vi "BeamTableEditor.vi"() -> ()   [LabVIEW 2021]
uses:
  D:/tmytek/Source/bbox-api/windows example/BBoxOne Series/LabVIEW/BBoxAPI.dll
  BBoxAPI.dll
  kernel32.dll
panel:
  in  "RX Beam Pattern":bool
  in  "RX beamId :\nRange from\n1 to 64":i32=1 min=1 max=64 step=1
  in  "RX_MIN_GAIN\nto\nRX_MAX_GAIN":dbl step=0.5
  in  "RX Theta \nRange from\n0 to 45":i32 min=0 max=45 step=1
  in  "RX Phi :\nRange from\n0 to 359":i32 min=0 max=359 step=1
  out "RX Store Beam Return":i32(ring) items=["OK"=0, "WARNING"=1, "ERROR"=2, "NO_RESPONSE"=3, "ERROR_GET_SN"=10, "ERROR_DEV_TYPE"=11, "ERROR_INIT_OBJECT"=12, "ERROR_DEV_NOT_INIT"=13, "ERROR_METHOD_NOT_FOUND"=14, "ERROR_REFLECTION"=15, "ERROR_POWER"=16, "ERROR_SCAN_NOT_FOUND"=17, "ERROR_UNMATCH_RETURN_TYPE"=18, "ERROR_NETWORK_NOT_INIT"=20, "ERROR_NETWORK_INIT"=21, "ERROR_NETWORK_CONNECT_TIMEOUT"=22, "ERROR_DISCONNECT"=23, "ERROR_SOCKET"=24, "ERROR_SEND_CMD"=25, "ERROR_RESP_CMD"=26, "ERROR_DEV_COUNT_ZERO"=30, "ERROR_DEV_DUMMY_FUNC"=31, "ERROR_CMD"=40, "ERROR_CMD_INIT"=41, "ERROR_BF_AAKIT"=100, "ERROR_BF_NO_AAKIT"=101, "ERROR_BF_CALI_PATH"=102, "ERROR_BF_BEAMXY"=103, "ERROR_BF_GEN"=104, "ERROR_BF_TRMODE"=105, "STATUS_BF_LOAD_CALI_INCOMPLTE"=106, "ERROR_BF_LOAD_CALI_PARSE_FAILED"=107, "ERROR_BF_UNLOAD_CALI"=108, "ERROR_BF_CALI_VERSION_UNSUPPORTED"=109, "ERROR_BF_CALI_DATA_NOT_FOUND"=110, "ERROR_FREQ_EQUATION"=250, "ERROR_PLO_CRC"=251, "WARNING_HARMONIC"=252, "ERROR_HARMONIC_BLOCK"=253, "ERROR_FW_UPGRADE_IP_INVALID"=300, "ERROR_FW_VERSION_NOT_SUPPORT"=301]
  out "getFrequencyList":string[](array[string])
  out "SN":string
  out "current state":i32
  out "ScanningDevice":string[](array[string])
  out "Target SN":string
  in  "Device SN":string="B00000000-00"
  out "SN_is_match":bool
  out "Init":i32(ring) items=["OK"=0, "WARNING"=1, "ERROR"=2, "NO_RESPONSE"=3, "ERROR_GET_SN"=10, "ERROR_DEV_TYPE"=11, "ERROR_INIT_OBJECT"=12, "ERROR_DEV_NOT_INIT"=13, "ERROR_METHOD_NOT_FOUND"=14, "ERROR_REFLECTION"=15, "ERROR_POWER"=16, "ERROR_SCAN_NOT_FOUND"=17, "ERROR_UNMATCH_RETURN_TYPE"=18, "ERROR_NETWORK_NOT_INIT"=20, "ERROR_NETWORK_INIT"=21, "ERROR_NETWORK_CONNECT_TIMEOUT"=22, "ERROR_DISCONNECT"=23, "ERROR_SOCKET"=24, "ERROR_SEND_CMD"=25, "ERROR_RESP_CMD"=26, "ERROR_DEV_COUNT_ZERO"=30, "ERROR_DEV_DUMMY_FUNC"=31, "ERROR_CMD"=40, "ERROR_CMD_INIT"=41, "ERROR_BF_AAKIT"=100, "ERROR_BF_NO_AAKIT"=101, "ERROR_BF_CALI_PATH"=102, "ERROR_BF_BEAMXY"=103, "ERROR_BF_GEN"=104, "ERROR_BF_TRMODE"=105, "STATUS_BF_LOAD_CALI_INCOMPLTE"=106, "ERROR_BF_LOAD_CALI_PARSE_FAILED"=107, "ERROR_BF_UNLOAD_CALI"=108, "ERROR_BF_CALI_VERSION_UNSUPPORTED"=109, "ERROR_BF_CALI_DATA_NOT_FOUND"=110, "ERROR_FREQ_EQUATION"=250, "ERROR_PLO_CRC"=251, "WARNING_HARMONIC"=252, "ERROR_HARMONIC_BLOCK"=253, "ERROR_FW_UPGRADE_IP_INVALID"=300, "ERROR_FW_VERSION_NOT_SUPPORT"=301]
  out "checkCaliTableLocation":bool
  out "Console Log":string
  in  "Target Freq Index":i32 min=1 max=2 step=1
  out "setOperatingFreq":i32(ring)=2 items=["OK"=0, "WARNING"=1, "ERROR"=2, "NO_RESPONSE"=3, "ERROR_GET_SN"=10, "ERROR_DEV_TYPE"=11, "ERROR_INIT_OBJECT"=12, "ERROR_DEV_NOT_INIT"=13, "ERROR_METHOD_NOT_FOUND"=14, "ERROR_REFLECTION"=15, "ERROR_POWER"=16, "ERROR_NETWORK_NOT_INIT"=20, "ERROR_NETWORK_INIT"=21, "ERROR_NETWORK_CONNECT_TIMEOUT"=22, "ERROR_DISCONNECT"=23, "ERROR_SOCKET"=24, "ERROR_SEND_CMD"=25, "ERROR_RESP_CMD"=26, "ERROR_DEV_COUNT_ZERO"=30, "ERROR_CMD"=40, "ERROR_CMD_INIT"=41, "ERROR_BF_AAKIT"=100, "ERROR_BF_NO_AAKIT"=101, "ERROR_BF_CALI_PATH"=102, "ERROR_BF_BEAMXY"=103, "ERROR_BF_GEN"=104, "ERROR_BF_TRMODE"=105, "STATUS_BF_LOAD_CALI_INCOMPLTE"=106, "ERROR_BF_LOAD_CALI_PARSE_FAILED"=107, "ERROR_FREQ_EQUATION"=250, "ERROR_PLO_CRC"=251, "WARNING_HARMONIC"=252, "ERROR_HARMONIC_BLOCK"=253]
  out "TX_MIN_GAIN":dbl
  out "TX_MAX_GAIN":dbl
  out "RX_MIN_GAIN":dbl
  out "RX_MAX_GAIN":dbl
  out "getAAKitList":string[](array[string])
  out "selectAAKit":i32(ring)=2 items=["OK"=0, "WARNING"=1, "ERROR"=2, "NO_RESPONSE"=3, "ERROR_GET_SN"=10, "ERROR_DEV_TYPE"=11, "ERROR_INIT_OBJECT"=12, "ERROR_DEV_NOT_INIT"=13, "ERROR_METHOD_NOT_FOUND"=14, "ERROR_REFLECTION"=15, "ERROR_POWER"=16, "ERROR_NETWORK_NOT_INIT"=20, "ERROR_NETWORK_INIT"=21, "ERROR_NETWORK_CONNECT_TIMEOUT"=22, "ERROR_DISCONNECT"=23, "ERROR_SOCKET"=24, "ERROR_SEND_CMD"=25, "ERROR_RESP_CMD"=26, "ERROR_DEV_COUNT_ZERO"=30, "ERROR_CMD"=40, "ERROR_CMD_INIT"=41, "ERROR_BF_AAKIT"=100, "ERROR_BF_NO_AAKIT"=101, "ERROR_BF_CALI_PATH"=102, "ERROR_BF_BEAMXY"=103, "ERROR_BF_GEN"=104, "ERROR_BF_TRMODE"=105, "STATUS_BF_LOAD_CALI_INCOMPLTE"=106, "ERROR_BF_LOAD_CALI_PARSE_FAILED"=107, "ERROR_FREQ_EQUATION"=250, "ERROR_PLO_CRC"=251, "WARNING_HARMONIC"=252, "ERROR_HARMONIC_BLOCK"=253]
  out "RX Beam Table":string[][](array[string])
  out "TX Beam Table":string[][](array[string])
  in  "Target AAKit Index":i32 min=1 max=2 step=1
  out "Target AAKit Name":string
  in  "TX beamId :\nRange from\n1 to 64":i32=1 min=1 max=64 step=1
  in  "TX_MIN_GAIN\nto\nTX_MAX_GAIN":dbl step=0.5
  in  "TX Theta \nRange from\n0 to 45":i32 min=0 max=45 step=1
  in  "TX Phi :\nRange from\n0 to 359":i32 min=0 max=359 step=1
  out "TX Store Beam Return":i32(ring) items=["OK"=0, "WARNING"=1, "ERROR"=2, "NO_RESPONSE"=3, "ERROR_GET_SN"=10, "ERROR_DEV_TYPE"=11, "ERROR_INIT_OBJECT"=12, "ERROR_DEV_NOT_INIT"=13, "ERROR_METHOD_NOT_FOUND"=14, "ERROR_REFLECTION"=15, "ERROR_POWER"=16, "ERROR_SCAN_NOT_FOUND"=17, "ERROR_UNMATCH_RETURN_TYPE"=18, "ERROR_NETWORK_NOT_INIT"=20, "ERROR_NETWORK_INIT"=21, "ERROR_NETWORK_CONNECT_TIMEOUT"=22, "ERROR_DISCONNECT"=23, "ERROR_SOCKET"=24, "ERROR_SEND_CMD"=25, "ERROR_RESP_CMD"=26, "ERROR_DEV_COUNT_ZERO"=30, "ERROR_DEV_DUMMY_FUNC"=31, "ERROR_CMD"=40, "ERROR_CMD_INIT"=41, "ERROR_BF_AAKIT"=100, "ERROR_BF_NO_AAKIT"=101, "ERROR_BF_CALI_PATH"=102, "ERROR_BF_BEAMXY"=103, "ERROR_BF_GEN"=104, "ERROR_BF_TRMODE"=105, "STATUS_BF_LOAD_CALI_INCOMPLTE"=106, "ERROR_BF_LOAD_CALI_PARSE_FAILED"=107, "ERROR_BF_UNLOAD_CALI"=108, "ERROR_BF_CALI_VERSION_UNSUPPORTED"=109, "ERROR_BF_CALI_DATA_NOT_FOUND"=110, "ERROR_FREQ_EQUATION"=250, "ERROR_PLO_CRC"=251, "WARNING_HARMONIC"=252, "ERROR_HARMONIC_BLOCK"=253, "ERROR_FW_UPGRADE_IP_INVALID"=300, "ERROR_FW_VERSION_NOT_SUPPORT"=301]
  in  "Program Stop":bool
  in  "TX Beam Pattern":bool
  out "Exists Table Filenames":string[](array[string])
  out "Get Current Working Directory":path
  in  "Set Current Working Directory":path
  in  "Start":bool
  # "Notice:\n\n1.  User can directly edit the beam settings (beamId, mode, db, theta, phi) and run the program to store beam pattern.\n\n     1.1 Store beam pattern and then read all beam patterns to GUI.\n\n\n2. Beam gain range definition is as below\n\n      2.1 Dynamic range of TX mode contains TX_MIN_GAIN and TX_MAX_GAIN read from calibration table.\n\n      2.2 TX beam gain setting must less than or equal to TX_MAX_GAIN and larger than or equal to TX_MIN_GAIN.\n\n      2.3 Dynamic range of RX mode contains RX_MIN_GAIN and RX_MAX_GAIN read from the calibration table.\n\n      2.4 RX beam gain setting must less than or equal to RX_MAX_GAIN and larger than or equal to RX_MIN_GAIN.\n\n\n3. Beam Id range is from 1 to 64.\n\n\n4. TX mode equals to 1 and RX mode equals to 2.\n\n\n5. Theta range is  from 0 to 45.\n\n\n6. Phi range is from 0 to 359.\n\n\n7. The right side beam tables  are readonly.\n\n     7.1 The  table column definition is [ beamId, mode, db, theta, phi ]"
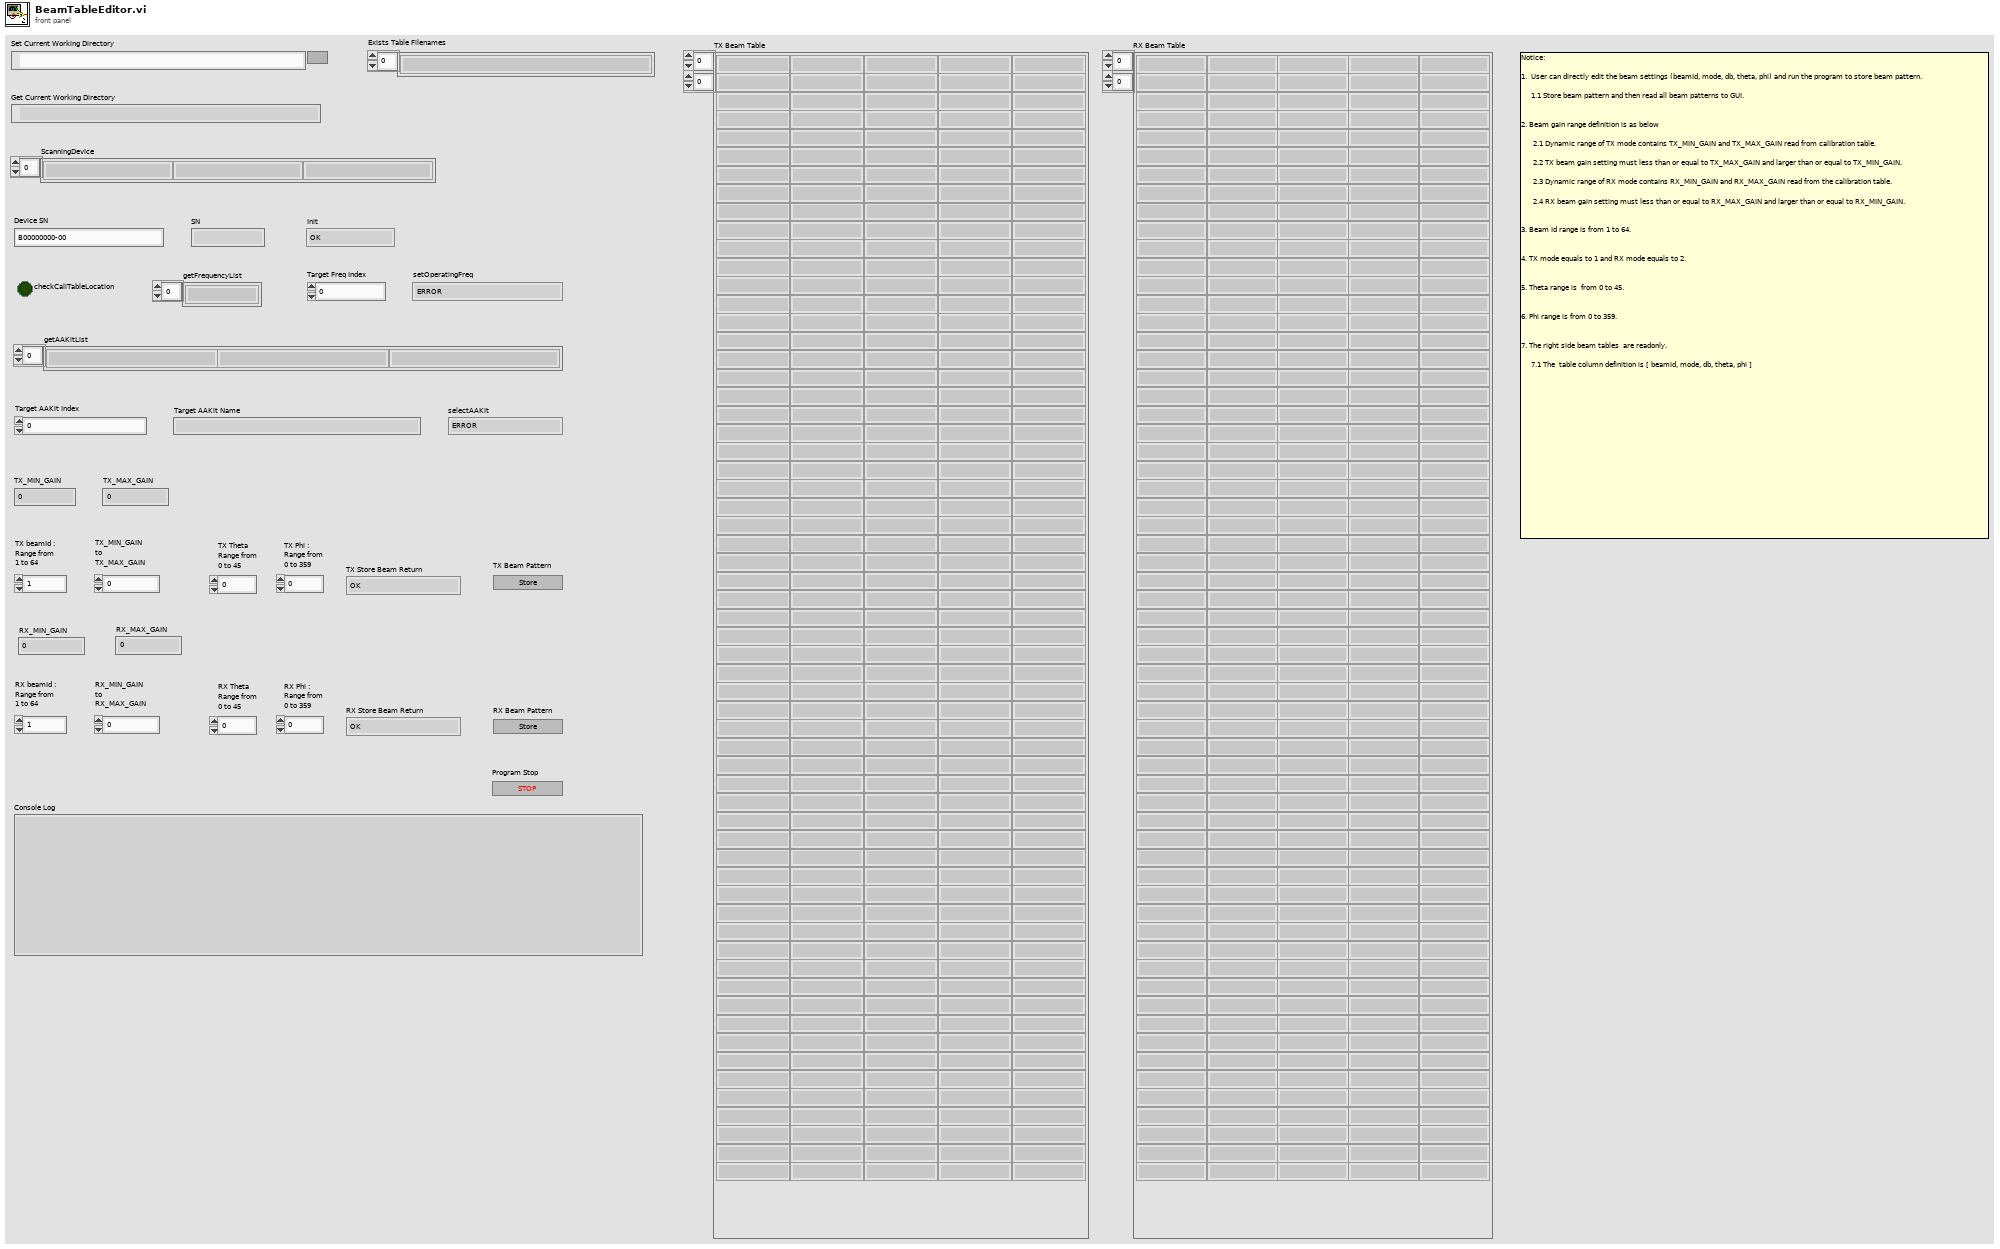
[diagram p1: front panel]
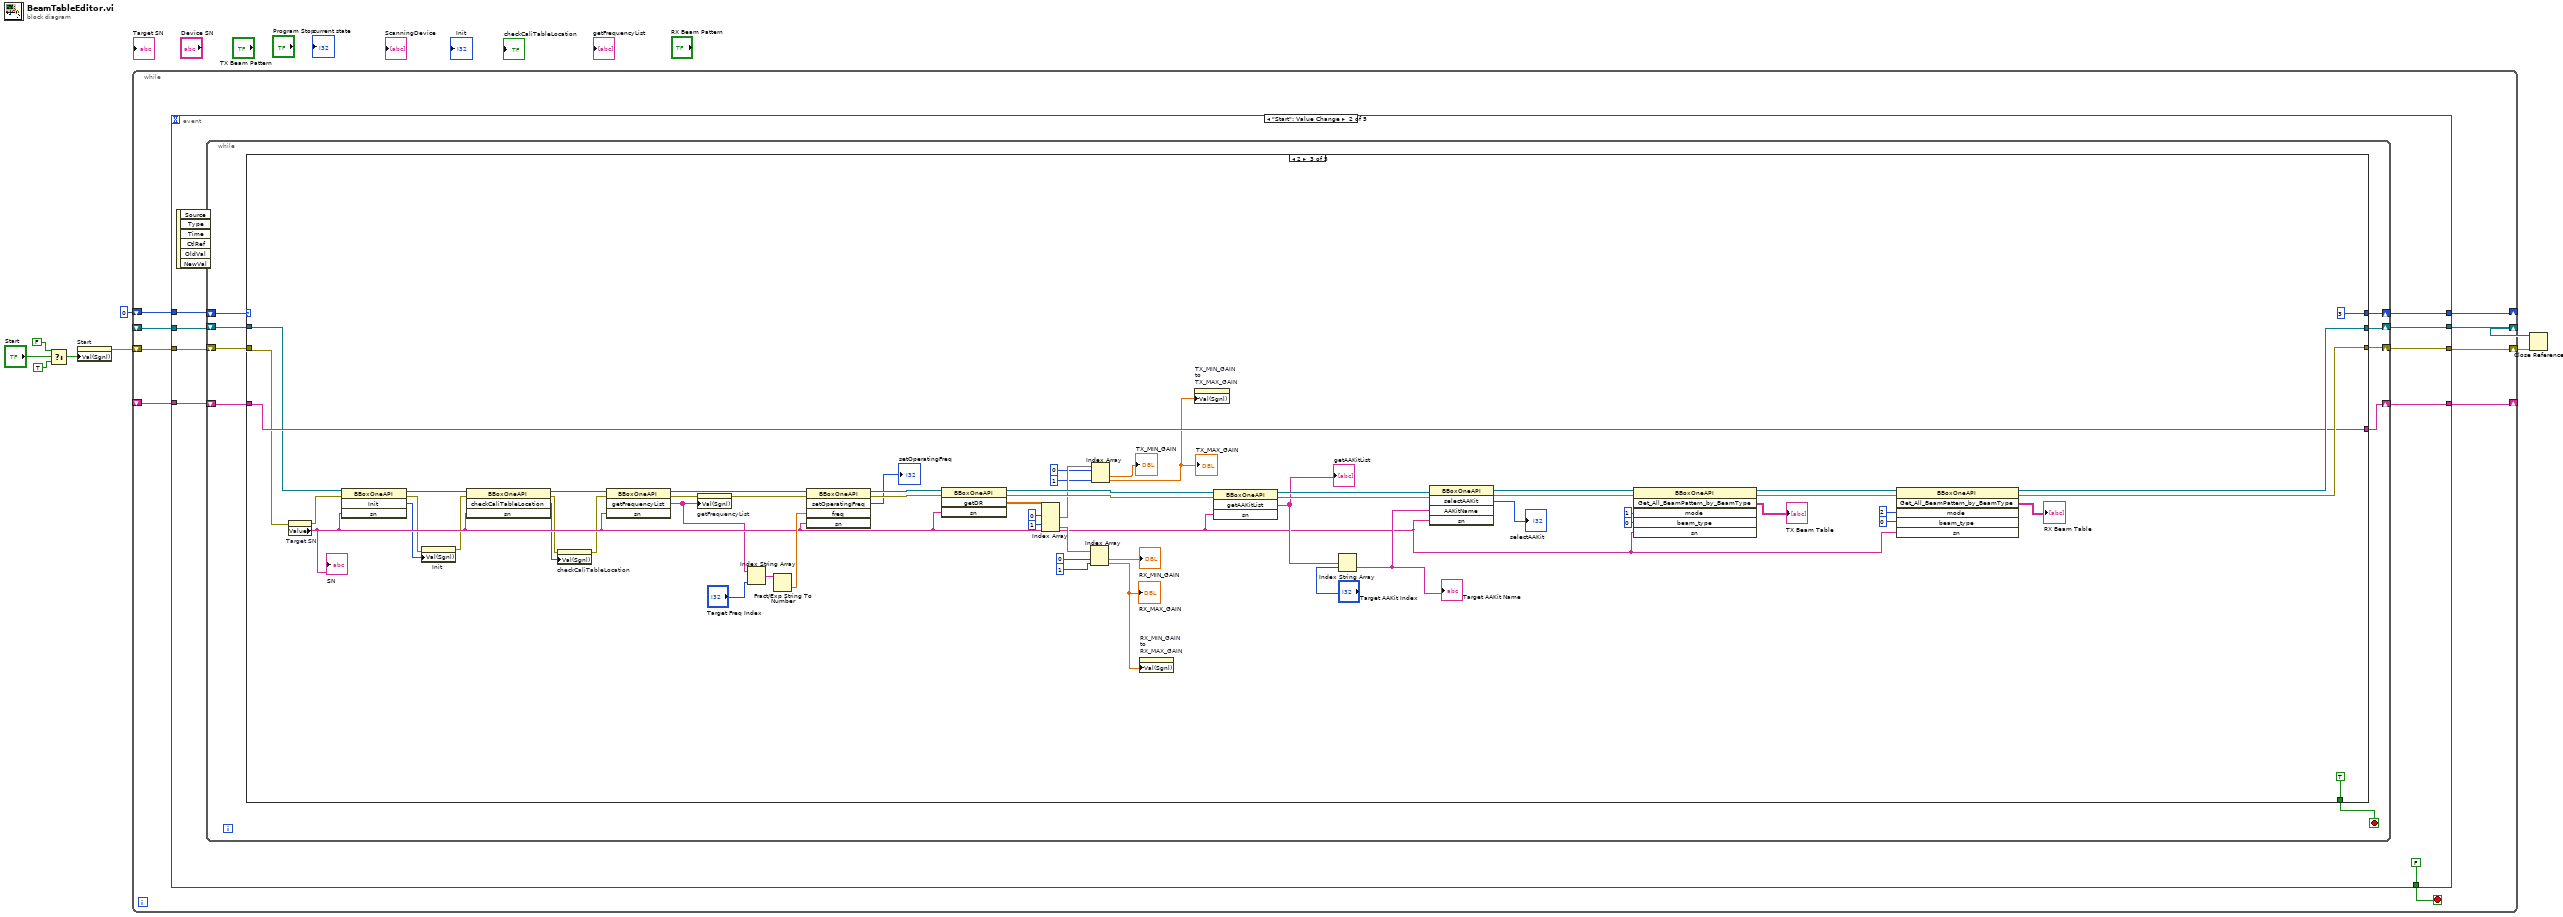
[diagram p0: block diagram]
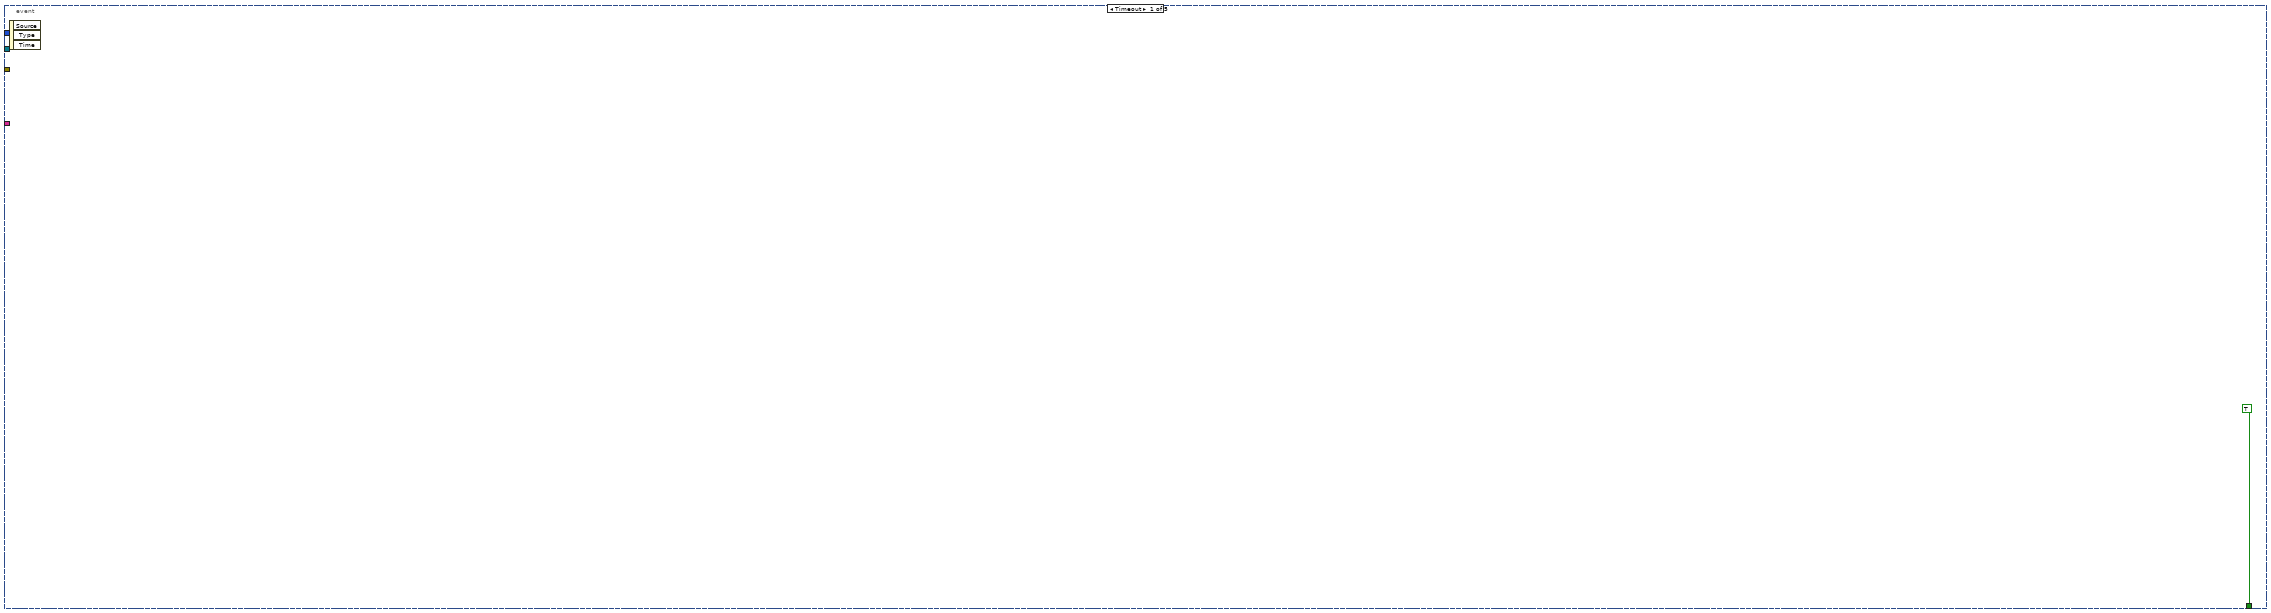
[diagram p2: hidden frame]
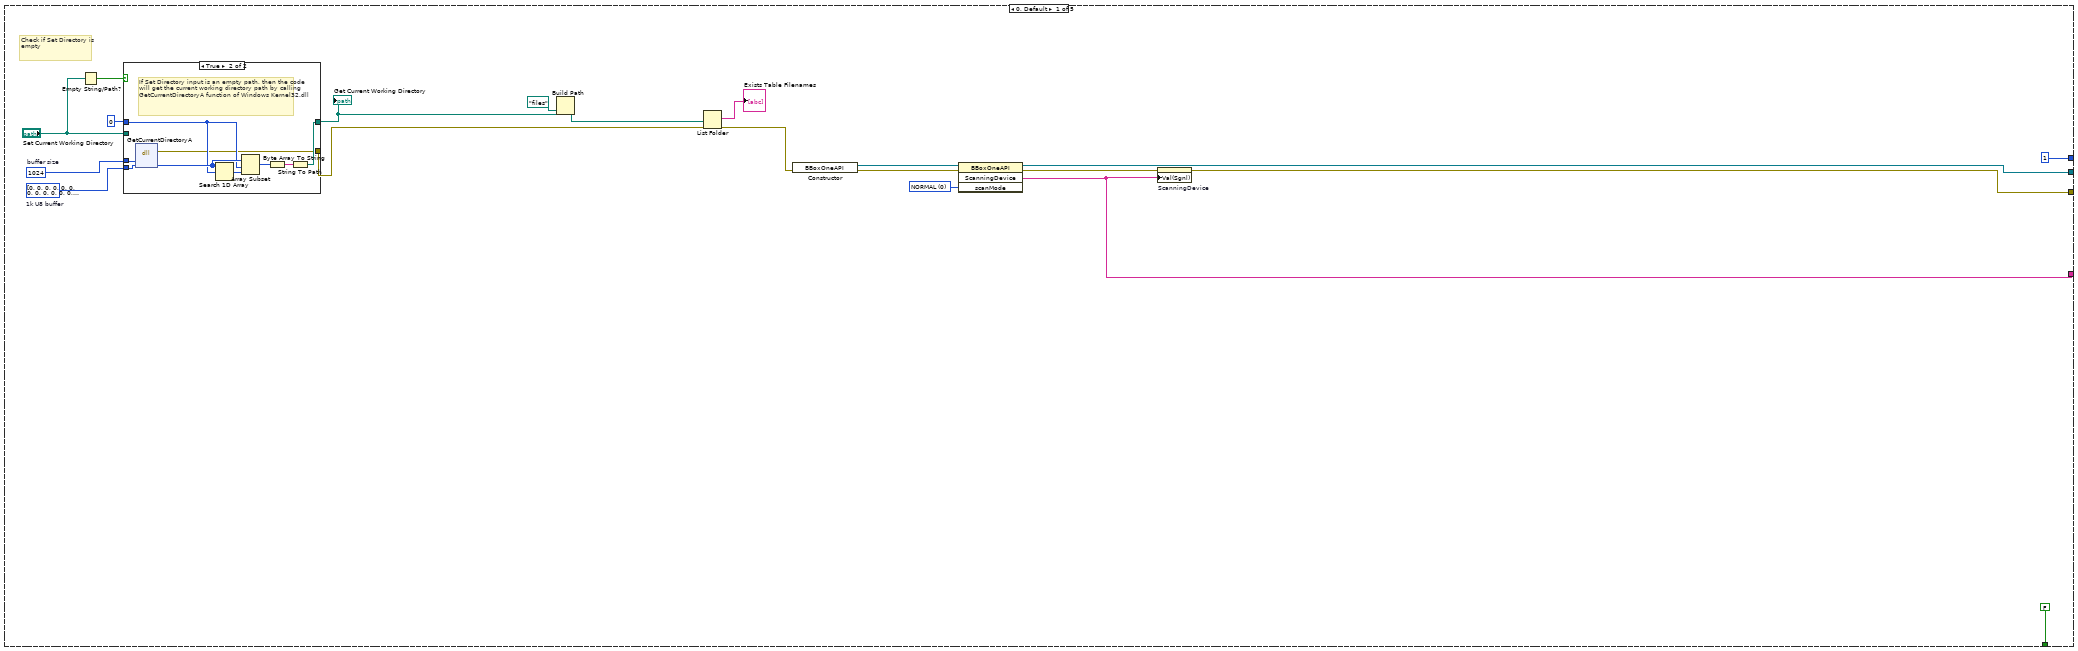
[diagram p3: hidden frame]
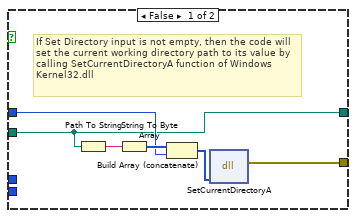
[diagram p4: hidden frame]
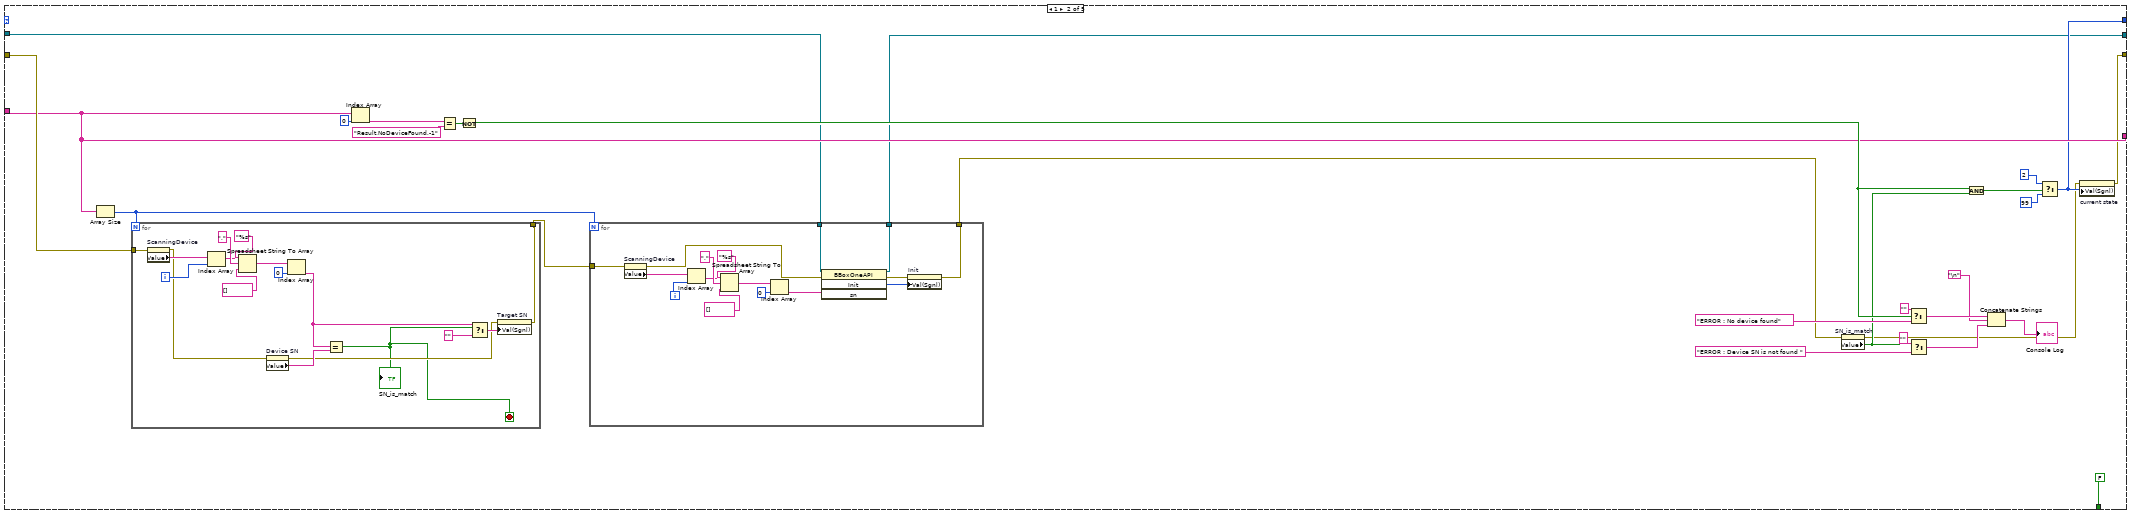
[diagram p5: hidden frame]
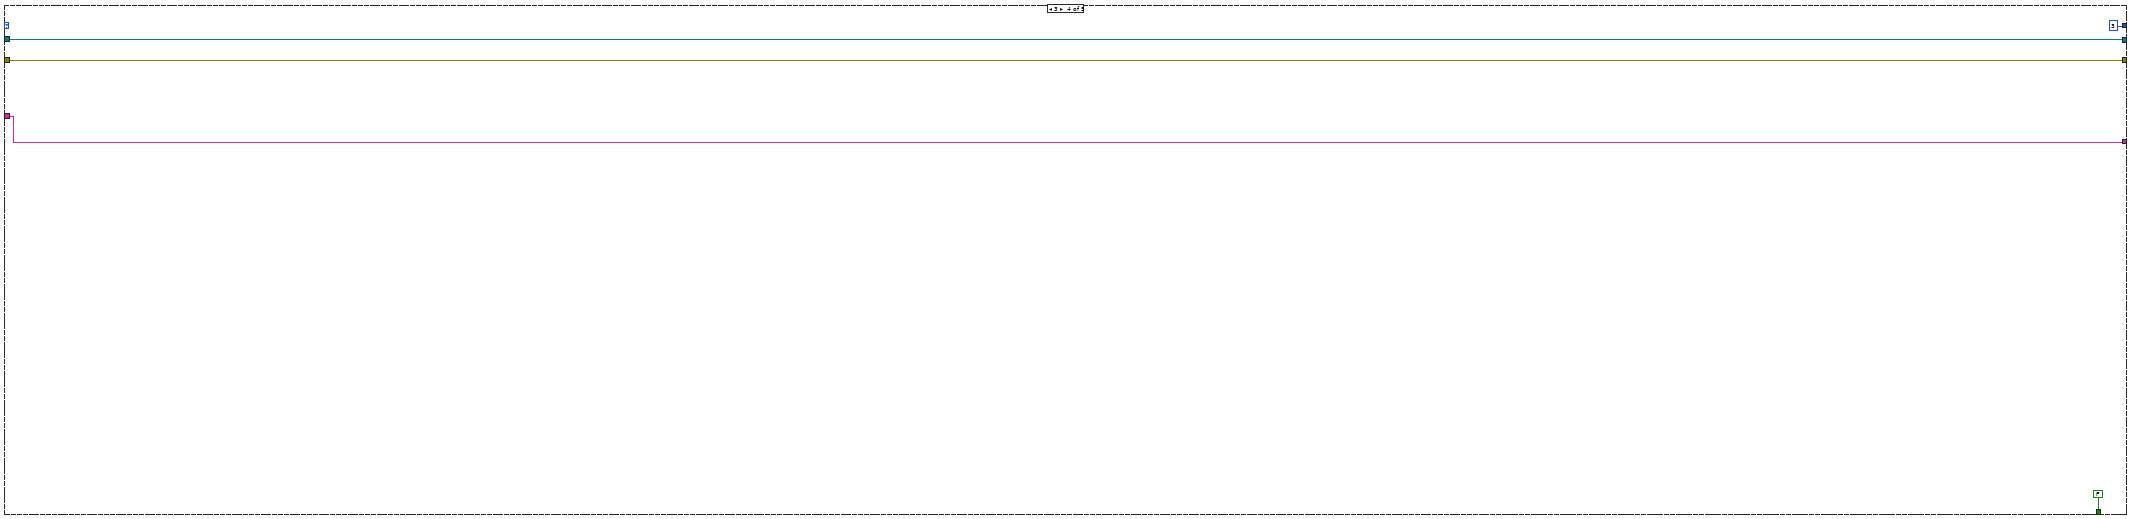
[diagram p6: hidden frame]
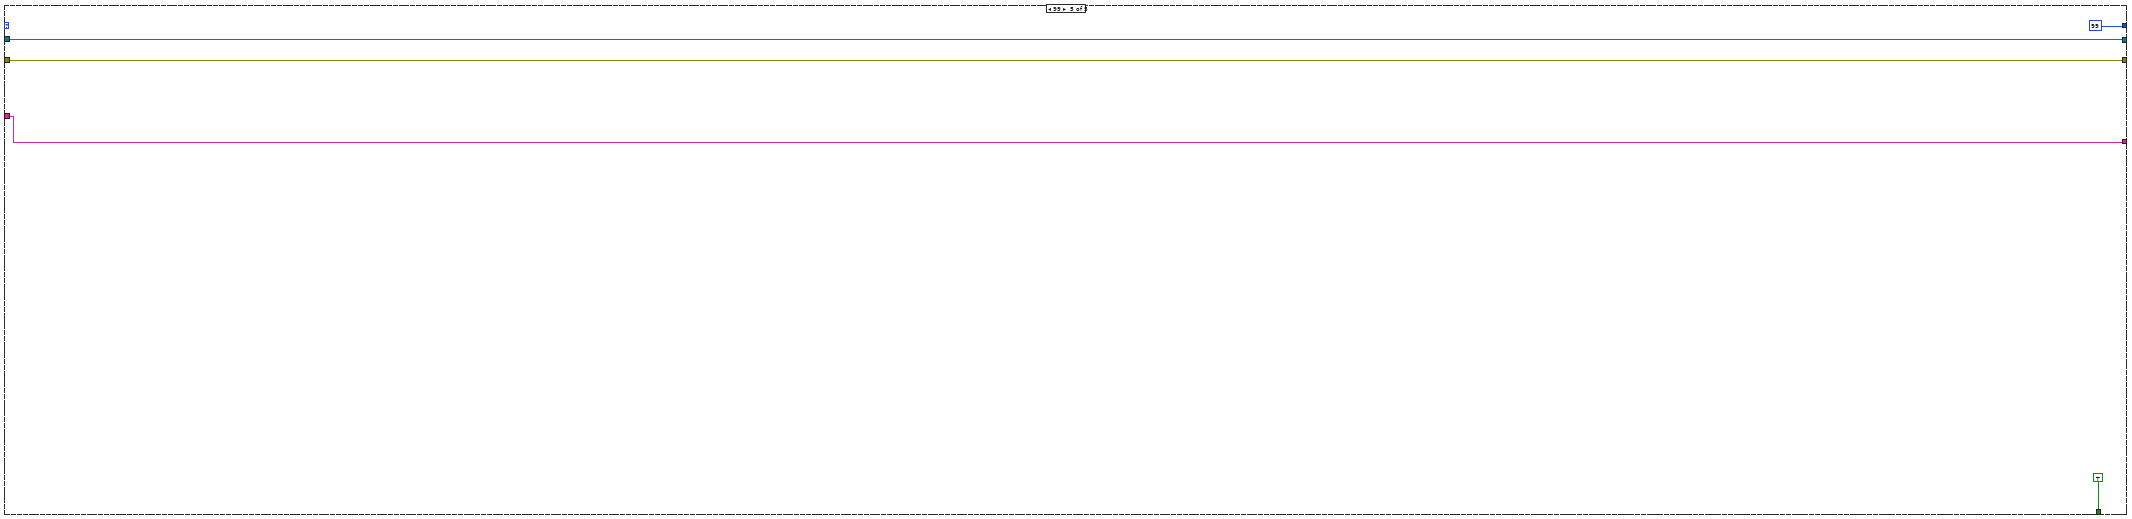
[diagram p7: hidden frame]
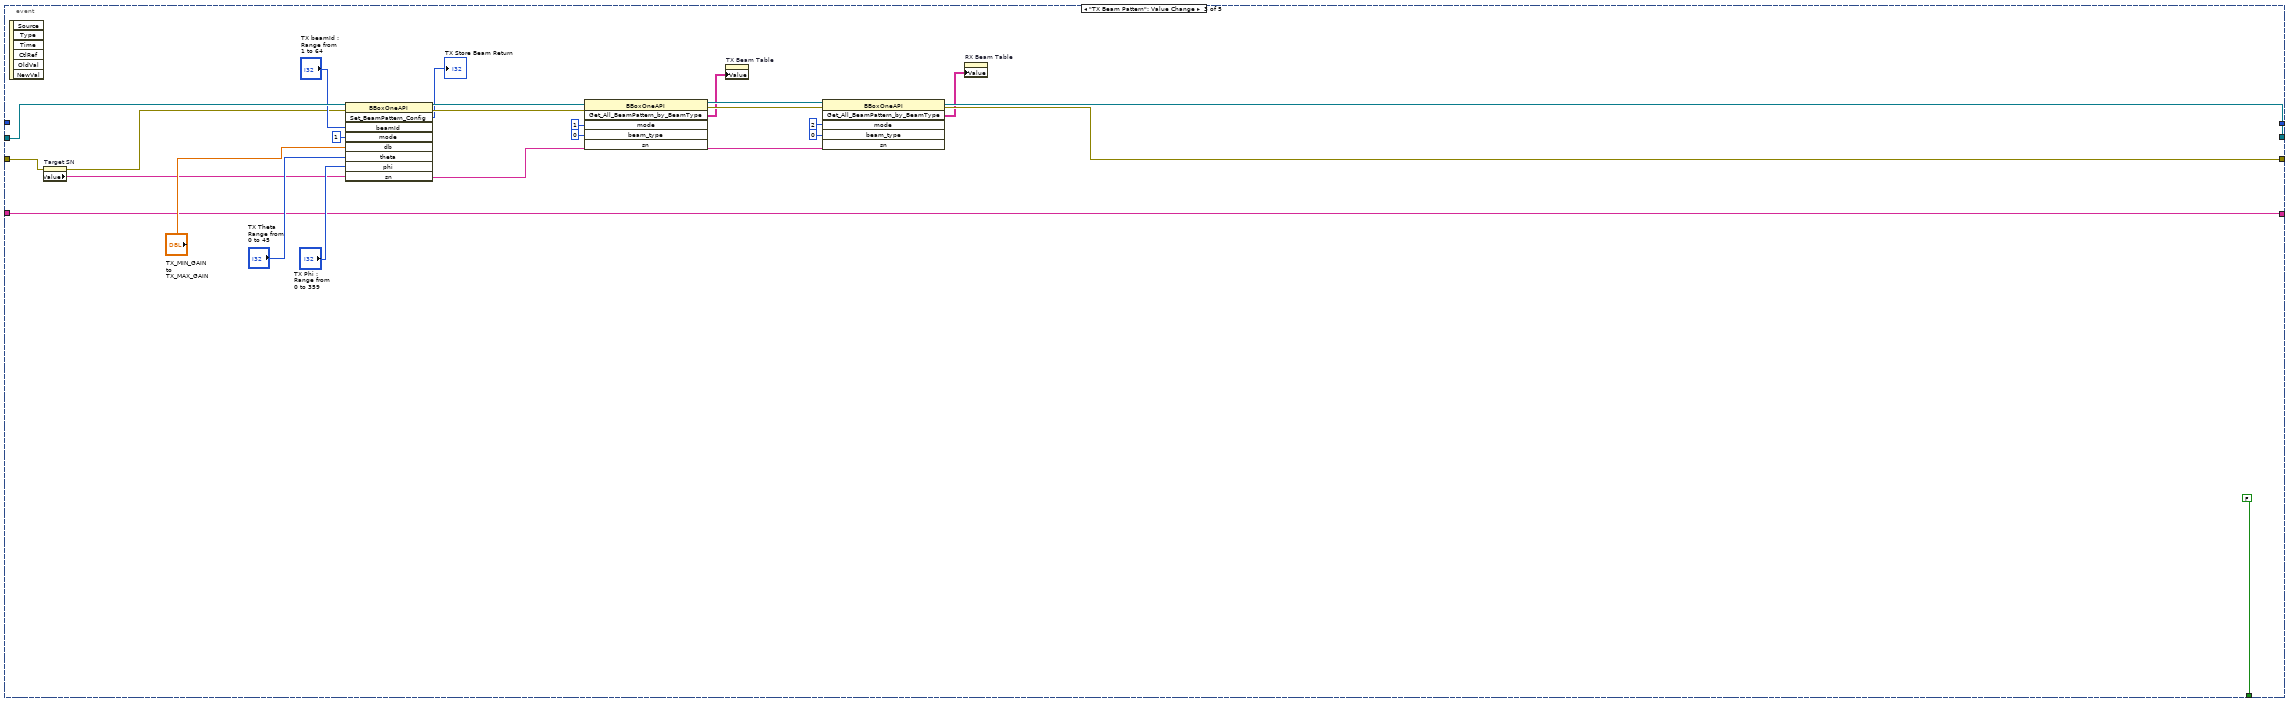
[diagram p8: hidden frame]
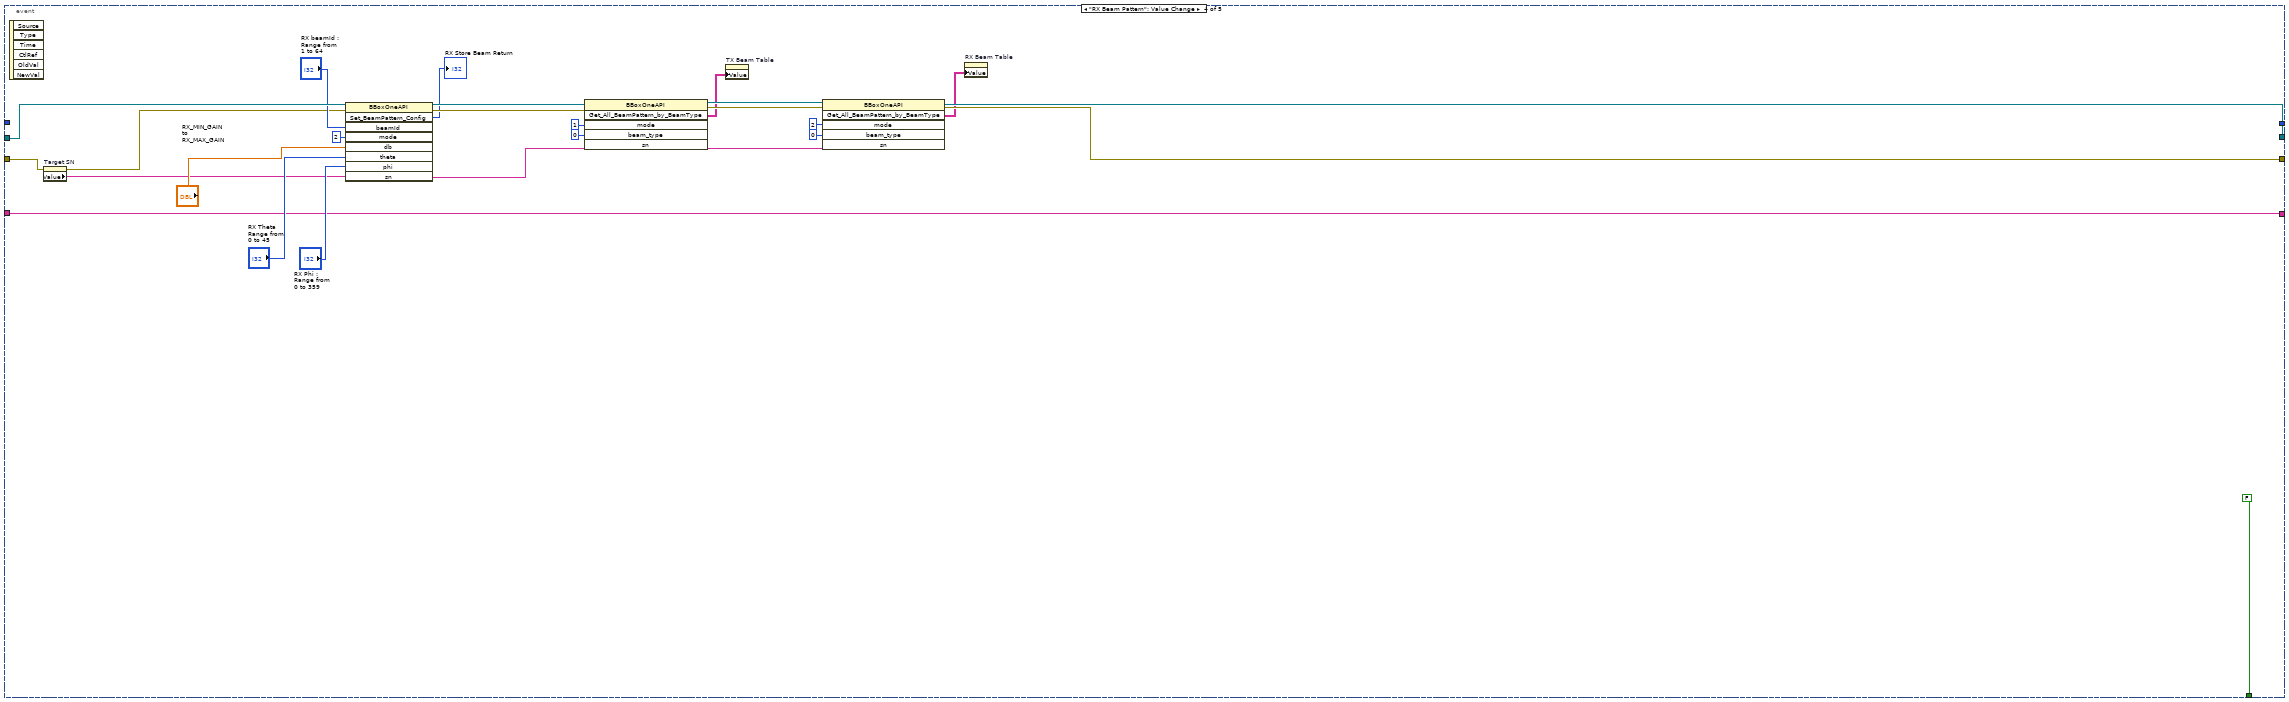
[diagram p9: hidden frame]
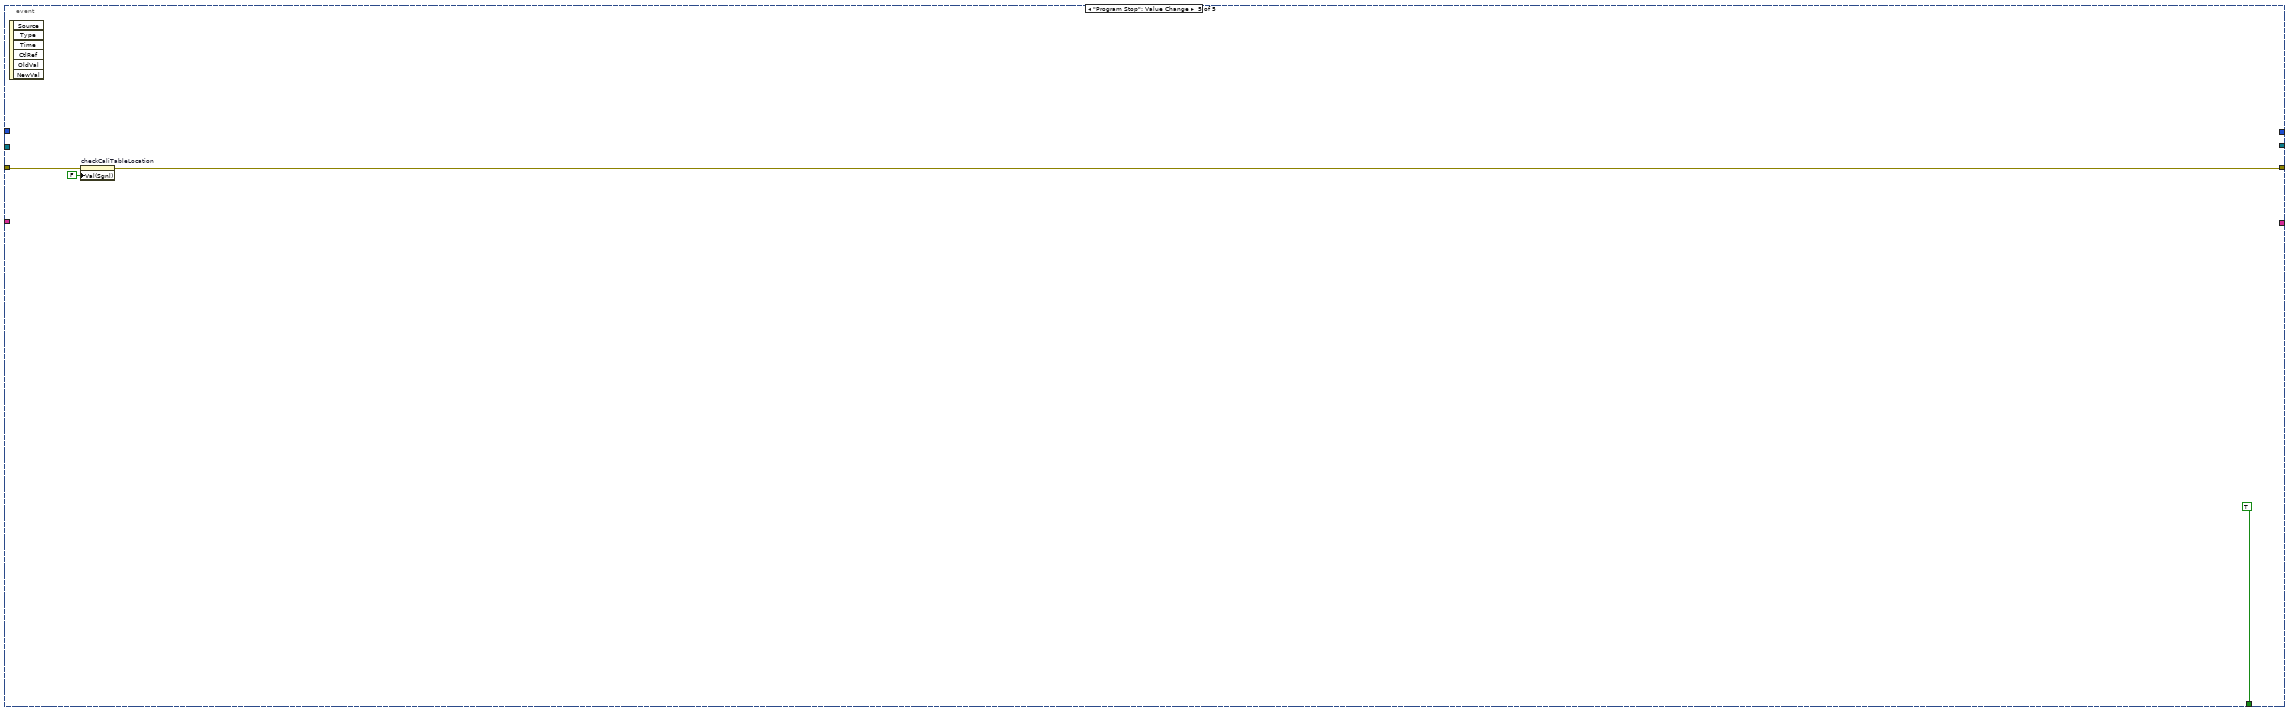
[diagram p10: hidden frame]
diagram:
  n1 = Select(t=FALSE, s="Start", f=TRUE) -> (s? t:f=w6:bool)
  n2 = property on="Start" class="Bool (strict)"("Val(Sgnl)"=w6) -> (error out=w3:errorcluster)  [unwired: 2 in, 1 out]
  n3 = while {
    shift-right: [w16] -> w8
    shift-left: _ -> [w14]
    shift-right: [w15] -> w7
    shift-left: w3 -> [w13]
    shift-right: [w12] -> _
    shift-left: _ -> [w11]
    shift-right: [w10] -> _
    shift-left: 0 -> [w9]
    stop <- w17 stop-if-true
    n4 = event shown="[1] \"Start\": Value Change" {
      selector: _ -> [_ _ _ _ _]
      dyn-events: _ -> [_ _ _ _ _]
      timeout: _ -> [_ _ _ _ _]
      tunnel: [TRUE FALSE FALSE FALSE TRUE] -> w17
      tunnel: [_ w27 w214 w238 _] -> w16
      tunnel: [_ w26 w213 w237 w249] -> w15
      tunnel: w14 -> [_ w25 w223 w247 _]
      tunnel: w13 -> [_ w24 w203 w227 w251]
      tunnel: [_ w22 w205 w229 _] -> w12
      tunnel: w11 -> [_ w21 w205 w229 _]
      tunnel: [_ w20 _ _ _] -> w10
      tunnel: w9 -> [_ w19 _ _ _]
      event Timeout {
        n5 = event-data() -> ()  [unwired: 1 in, 3 out]
      }
      event "Start": Value Change {
        n6 = event-data() -> ()  [unwired: 1 in, 6 out]
        n7 = while {
          shift-right: [w36] -> w20
          shift-left: w19 -> [w28]
          shift-right: [w35] -> w27
          shift-left: w25 -> [w33]
          shift-right: [w34] -> w26
          shift-left: w24 -> [w32]
          shift-right: [w30] -> w22
          shift-left: w21 -> [w29]
          stop <- w31 stop-if-true
          n8 = case shown="2" w28 {
            tunnel: [w37 w81 w156 w194 w198] -> w34
            tunnel: [w41 w73 w157 w195 w197] -> w35
            tunnel: [1 w82 3 3 99] -> w36
            tunnel: [FALSE FALSE TRUE FALSE TRUE] -> w31
            tunnel: w33 -> [_ w74 w146 w195 w197]
            tunnel: w32 -> [_ w84 w150 w194 w198]
            tunnel: [w39 w83 w154 w193 w196] -> w30
            tunnel: w29 -> [_ w83 w154 w193 w196]
            frame 0, Default {
              w51 = 1024  # buffer size
              w56 = 0 items=["NORMAL", "FAST"] ("scanMode")
              w50 = u8[] [0, 0, 0, 0, 0, 0, 0, 0, 0, 0, 0, 0, 0, 0, 0, 0, 0, 0, 0, 0, 0, 0, 0, 0, 0, 0, 0, 0, 0, 0, 0, 0, 0, 0, 0, 0, 0, 0, 0, 0, 0, 0, 0, 0, 0, 0, 0, 0, 0, 0, 0, 0, 0, 0, 0, 0, 0, 0, 0, 0, 0, 0, 0, 0, 0, 0, 0, 0, 0, 0, 0, 0, 0, 0, 0, 0, 0, 0, 0, 0, 0, 0, 0, 0, 0, 0, 0, 0, 0, 0, 0, 0, 0, 0, 0, 0, 0, 0, 0, 0, 0, 0, 0, 0, 0, 0, 0, 0, 0, 0, 0, 0, 0, 0, 0, 0, 0, 0, 0, 0, 0, 0, 0, 0, 0, 0, 0, 0, 0, 0, 0, 0, 0, 0, 0, 0, 0, 0, 0, 0, 0, 0, 0, 0, 0, 0, 0, 0, 0, 0, 0, 0, 0, 0, 0, 0, 0, 0, 0, 0, 0, 0, 0, 0, 0, 0, 0, 0, 0, 0, 0, 0, 0, 0, 0, 0, 0, 0, 0, 0, 0, 0, 0, 0, 0, 0, 0, 0, 0, 0, 0, 0, 0, 0, 0, 0, 0, 0, 0, 0, 0, 0, 0, 0, 0, 0, 0, 0, 0, 0, 0, 0, 0, 0, 0, 0, 0, 0, 0, 0, 0, 0, 0, 0, 0, 0, 0, 0, 0, 0, 0, 0, 0, 0, 0, 0, 0, 0, 0, 0, 0, 0, 0, 0, 0, 0, 0, 0, 0, 0, 0, 0, 0, 0, 0, 0, 0, 0, 0, 0, 0, 0, 0, 0, 0, 0, 0, 0, 0, 0, 0, 0, 0, 0, 0, 0, 0, 0, 0, 0, 0, 0, 0, 0, 0, 0, 0, 0, 0, 0, 0, 0, 0, 0, 0, 0, 0, 0, 0, 0, 0, 0, 0, 0, 0, 0, 0, 0, 0, 0, 0, 0, 0, 0, 0, 0, 0, 0, 0, 0, 0, 0, 0, 0, 0, 0, 0, 0, 0, 0, 0, 0, 0, 0, 0, 0, 0, 0, 0, 0, 0, 0, 0, 0, 0, 0, 0, 0, 0, 0, 0, 0, 0, 0, 0, 0, 0, 0, 0, 0, 0, 0, 0, 0, 0, 0, 0, 0, 0, 0, 0, 0, 0, 0, 0, 0, 0, 0, 0, 0, 0, 0, 0, 0, 0, 0, 0, 0, 0, 0, 0, 0, 0, 0, 0, 0, 0, 0, 0, 0, 0, 0, 0, 0, 0, 0, 0, 0, 0, 0, 0, 0, 0, 0, 0, 0, 0, 0, 0, 0, 0, 0, 0, 0, 0, 0, 0, 0, 0, 0, 0, 0, 0, 0, 0, 0, 0, 0, 0, 0, 0, 0, 0, 0, 0, 0, 0, 0, 0, 0, 0, 0, 0, 0, 0, 0, 0, 0, 0, 0, 0, 0, 0, 0, 0, 0, 0, 0, 0, 0, 0, 0, 0, 0, 0, 0, 0, 0, 0, 0, 0, 0, 0, 0, 0, 0, 0, 0, 0, 0, 0, 0, 0, 0, 0, 0, 0, 0, 0, 0, 0, 0, 0, 0, 0, 0, 0, 0, 0, 0, 0, 0, 0, 0, 0, 0, 0, 0, 0, 0, 0, 0, 0, 0, 0, 0, 0, 0, 0, 0, 0, 0, 0, 0, 0, 0, 0, 0, 0, 0, 0, 0, 0, 0, 0, 0, 0, 0, 0, 0, 0, 0, 0, 0, 0, 0, 0, 0, 0, 0, 0, 0, 0, 0, 0, 0, 0, 0, 0, 0, 0, 0, 0, 0, 0, 0, 0, 0, 0, 0, 0, 0, 0, 0, 0, 0, 0, 0, 0, 0, 0, 0, 0, 0, 0, 0, 0, 0, 0, 0, 0, 0, 0, 0, 0, 0, 0, 0, 0, 0, 0, 0, 0, 0, 0, 0, 0, 0, 0, 0, 0, 0, 0, 0, 0, 0, 0, 0, 0, 0, 0, 0, 0, 0, 0, 0, 0, 0, 0, 0, 0, 0, 0, 0, 0, 0, 0, 0, 0, 0, 0, 0, 0, 0, 0, 0, 0, 0, 0, 0, 0, 0, 0, 0, 0, 0, 0, 0, 0, 0, 0, 0, 0, 0, 0, 0, 0, 0, 0, 0, 0, 0, 0, 0, 0, 0, 0, 0, 0, 0, 0, 0, 0, 0, 0, 0, 0, 0, 0, 0, 0, 0, 0, 0, 0, 0, 0, 0, 0, 0, 0, 0, 0, 0, 0, 0, 0, 0, 0, 0, 0, 0, 0, 0, 0, 0, 0, 0, 0, 0, 0, 0, 0, 0, 0, 0, 0, 0, 0, 0, 0, 0, 0, 0, 0, 0, 0, 0, 0, 0, 0, 0, 0, 0, 0, 0, 0, 0, 0, 0, 0, 0, 0, 0, 0, 0, 0, 0, 0, 0, 0, 0, 0, 0, 0, 0, 0, 0, 0, 0, 0, 0, 0, 0, 0, 0, 0, 0, 0, 0, 0, 0, 0, 0, 0, 0, 0, 0, 0, 0, 0, 0, 0, 0, 0, 0, 0, 0, 0, 0, 0, 0, 0, 0, 0, 0, 0, 0, 0, 0, 0, 0, 0, 0, 0, 0, 0, 0, 0, 0, 0, 0, 0, 0, 0, 0, 0, 0, 0, 0, 0, 0, 0, 0, 0, 0, 0, 0, 0, 0, 0, 0, 0, 0, 0, 0, 0, 0, 0, 0, 0, 0, 0, 0, 0, 0, 0, 0, 0, 0, 0, 0, 0, 0, 0, 0, 0, 0, 0, 0, 0, 0, 0, 0, 0, 0, 0, 0, 0, 0, 0, 0, 0, 0, 0, 0, 0, 0, 0, 0, 0, 0, 0, 0, 0, 0, 0, 0, 0, 0, 0, 0, 0, 0, 0, 0, 0, 0, 0, 0, 0, 0, 0, 0, 0, 0, 0, 0, 0, 0, 0, 0, 0, 0, 0, 0, 0, 0, 0, 0, 0, 0, 0, 0, 0, 0, 0, 0, 0, 0, 0, 0, 0, 0, 0, 0, 0, 0, 0, 0, 0, 0, 0, 0, 0, 0, 0, 0, 0, 0, 0, 0, 0, 0, 0, 0, 0, 0, 0, 0, 0, 0, 0, 0, 0, 0, 0, 0, 0, 0, 0, 0, 0, 0, 0, 0, 0, 0, 0, 0, 0, 0, 0, 0, 0, 0, 0, 0, 0, 0, 0, 0, 0, 0, 0, 0, 0, 0, 0, 0, 0, 0, 0, 0]  # 1k U8 buffer
              # "Check if Set Directory is empty"
              n9 = Empty String/Path?(string/path="Set Current Working Directory") -> (empty?=w52:bool)
              n10 = case shown="True" w52 {
                tunnel: "Set Current Working Directory" -> [w58 _]
                tunnel: u8 0 -> [w60 w67]
                tunnel: w51 -> [_ w66]
                tunnel: w50 -> [_ w65]
                tunnel: [w58 w64] -> w45
                tunnel: [w57 w63] -> w44
                frame False {
                  # "If Set Directory input is not empty, then the code will set the current working directory path to its value by calling SetCurrentDirectoryA function of Windows Kernel32.dll"
                  n11 = Path To String(path=w58) -> (string=w59:string)
                  n12 = String To Byte Array(string=w59) -> (unsigned byte array=w62:u8[])
                  n13 = Build Array (concatenate)(w62, w60) -> (w61:u8[])
                  n14 = dll-call lib="Kernel32.dll" fn="SetCurrentDirectoryA" label="Kernel32.dll - \nSetCurrentDirectoryA"("lpPathName"=w61) -> (error out=w57:errorcluster)  [unwired: 4 in, 2 out]
                }
                frame True {
                  # "If Set Directory input is an empty path, then the code will get the current working directory path by calling GetCurrentDirectoryA function of Windows Kernel32.dll"
                  n15 = dll-call lib="kernel32.dll" fn="GetCurrentDirectoryA" label="Kernel32.dll - \nGetCurrentDirectoryA"("nBufferLength"=w66, "lpBuffer"=w65) -> (error out=w63:errorcluster, "lpBuffer"=w70:u8[])  [unwired: 4 in, 2 out]
                  n16 = Search 1D Array(1D array=w70, element=w67) -> (index of element=w71:i32)  [unwired: 1 out]
                  n17 = Array Subset(array=w70, index=w67, length=w71) -> (w68:u8[])
                  n18 = Byte Array To String(unsigned byte array=w68) -> (string=w69:string)
                  n19 = String To Path(string=w69) -> (path=w64:path)
                }
              }
              "Get Current Working Directory" <- w45
              n20 = Build Path(base path=w45, name or relative path=path "files") -> (appended path=w46:path)
              n21 = List Folder(path=w46, error in=w44) -> (filenames=→"Exists Table Filenames":string[], error out=w43:errorcluster)  [unwired: 2 in, 2 out]
              n22 = constructor class="BBoxOneAPI"(error in=w43) -> (reference out=w55:refnum<k24>, error out=w54:errorcluster)  [unwired: 2 in, 1 out]
              n23 = invoke class="BBoxOneAPI" method="ScanningDevice"(reference=w55, error in=w54, "scanMode"=w56) -> (reference out=w41:refnum<k24>, error out=w38:errorcluster, "ScanningDevice"=w39:string[])  [unwired: 1 in, 1 out]
              n24 = property on="ScanningDevice" class="Arr (strict)"(error in=w38, "Val(Sgnl)"=w39) -> (error out=w37:errorcluster)  [unwired: 1 in, 1 out]
            }
            frame 1 {
              n25 = Array Size(array=w83) -> (size(s)=w77:i32)
              n26 = for {
                N: w77 -> [_]
                tunnel: [w121] -> w76
                tunnel: w84 -> [w124]
                i -> [w127]
                stop <- w116 stop-if-true
                n27 = property on="ScanningDevice" class="Arr (strict)"(error in=w124) -> (error out=w119:errorcluster, "Value"=w123:string[])  [unwired: 1 in, 1 out]
                n28 = Index Array(array=w123, index=w127) -> (element=w130:string)
                n29 = Spreadsheet String To Array(delimiter (Tab)=",", format string="%s", spreadsheet string=w130, array type (2D Dbl)=string[] []) -> (array=w126:string[])
                n30 = property on="Device SN" class="Str"(error in=w119) -> (error out=w118:errorcluster, "Value"=w120:string)  [unwired: 1 in, 1 out]
                n31 = Index Array(array=w126, index=0) -> (element=w117:string)
                n32 = Equal?(x=w117, y=w120) -> (x = y?=w116:bool)
                "SN_is_match" <- w116
                n33 = Select(t=w117, s=w116, f="") -> (s? t:f=w122:string)
                n34 = property on="Target SN" class="Str"(error in=w118, "Val(Sgnl)"=w122) -> (error out=w121:errorcluster)  [unwired: 1 in, 1 out]
              }
              n35 = Index Array(array=w83, index=0) -> (element=w85:string)
              n36 = Equal?(x=w85, y="Result,NoDeviceFound,-1") -> (x = y?=w95:bool)
              n37 = Not(x=w95) -> (.not. x?=w90:bool)
              n38 = for {
                N: w77 -> [_]
                tunnel: w76 -> [w107]
                tunnel: [w100] -> w75
                tunnel: w74 -> [w104]
                tunnel: [w103] -> w73
                i -> [w109]
                n39 = property on="ScanningDevice" class="Arr (strict)"(error in=w107) -> (error out=w105:errorcluster, "Value"=w108:string[])  [unwired: 1 in, 1 out]
                n40 = Index Array(array=w108, index=w109) -> (element=w113:string)
                n41 = Spreadsheet String To Array(delimiter (Tab)=",", format string="%s", spreadsheet string=w113, array type (2D Dbl)=string[] []) -> (array=w110:string[])
                n42 = Index Array(array=w110, index=0) -> (element=w106:string)
                n43 = invoke class="BBoxOneAPI" method="Init"(reference=w104, error in=w105, "sn"=w106) -> (reference out=w103:refnum<k24>, error out=w101:errorcluster, "Init"=w102:i32)  [unwired: 1 in, 1 out]
                n44 = property on="Init" class="Ring (strict)"(error in=w101, "Val(Sgnl)"=w102) -> (error out=w100:errorcluster)  [unwired: 1 in, 1 out]
              }
              n45 = property on="SN_is_match" class="Bool (strict)"(error in=w75) -> (error out=w72:errorcluster, "Value"=w79:bool)  [unwired: 1 in, 1 out]
              n46 = Select(t="" ("y"), s=w90, f="ERROR : No device found" ("y")) -> (s? t:f=w92:string)
              n47 = Select(t="" ("y"), s=w79, f="ERROR : Device SN is not found " ("y")) -> (s? t:f=w80:string)
              n48 = And(x=w90, y=w79) -> (x .and. y?=w78:bool)
              n49 = Concatenate Strings(w92, "\n", w80) -> (→"Console Log":string)
              n50 = Select(t=2, s=w78, f=99) -> (s? t:f=w82:i32)
              n51 = property on="current state" class="DigNum (strict)"(error in=w72, "Val(Sgnl)"=w82) -> (error out=w81:errorcluster)  [unwired: 1 in, 1 out]
            }
            frame 2 {
              n52 = property on="Target SN" class="Str"(error in=w150) -> (error out=w147:errorcluster, "Value"=w144:string)  [unwired: 1 in, 1 out]
              "SN" <- w144
              n53 = invoke class="BBoxOneAPI" method="Init"(reference=w146, error in=w147, "sn"=w144) -> (reference out=w145:refnum<k24>, error out=w142:errorcluster, "Init"=w143:i32)  [unwired: 1 in, 1 out]
              n54 = property on="Init" class="Ring (strict)"(error in=w142, "Val(Sgnl)"=w143) -> (error out=w141:errorcluster)  [unwired: 1 in, 1 out]
              n55 = invoke class="BBoxOneAPI" method="checkCaliTableLocation"(reference=w145, error in=w141, "sn"=w144) -> (reference out=w149:refnum<k24>, error out=w140:errorcluster, "checkCaliTableLocation"=w138:bool)  [unwired: 1 in, 1 out]
              n56 = property on="checkCaliTableLocation" class="Bool (strict)"(error in=w140, "Val(Sgnl)"=w138) -> (error out=w139:errorcluster)  [unwired: 1 in, 1 out]
              n57 = invoke class="BBoxOneAPI" method="getFrequencyList"(reference=w149, error in=w139, "sn"=w144) -> (reference out=w148:refnum<k24>, error out=w137:errorcluster, "getFrequencyList"=w135:string[])  [unwired: 1 in, 1 out]
              n58 = property on="getFrequencyList" class="Arr (strict)"(error in=w137, "Val(Sgnl)"=w135) -> (error out=w136:errorcluster)  [unwired: 1 in, 1 out]
              n59 = Index String Array(1:"Target Freq Index", 2:w135) -> (0:w153:string)  [unwired: 1 in]
              n60 = Fract/Exp String To Number(string=w153) -> (number=w151:dbl)  [unwired: 3 in, 1 out]
              n61 = invoke class="BBoxOneAPI" method="setOperatingFreq"(reference=w148, error in=w136, "freq"=w151, "sn"=w144) -> (reference out=w180:refnum<k24>, error out=w179:errorcluster, "setOperatingFreq"=→"setOperatingFreq":i32)  [unwired: 1 in, 2 out]
              n62 = invoke class="BBoxOneAPI" method="getDR"(reference=w180, error in=w179, "sn"=w144) -> (reference out=w178:refnum<k24>, error out=w177:errorcluster, "getDR"=w176:dbl[][])  [unwired: 1 in, 1 out]
              n63 = Index Array(array=w176, index (row) #1=0 ("index (row)"), index (row) #2=1 ("index (row)")) -> (element #1=w173:dbl[], element #2=w170:dbl[])  [unwired: 2 in]
              n64 = Index Array(array=w170, index #1=0 ("index"), index #2=1 ("index")) -> (element #1=→"RX_MIN_GAIN":dbl, element #2=w133:dbl)
              "RX_MAX_GAIN" <- w133
              n65 = Index Array(array=w173, index #1=0 ("index"), index #2=1 ("index")) -> (element #1=→"TX_MIN_GAIN":dbl, element #2=w134:dbl)
              "TX_MAX_GAIN" <- w134
              n66 = property on="RX_MIN_GAIN\nto\nRX_MAX_GAIN" class="DigNum (strict)"("Val(Sgnl)"=w133) -> ()  [unwired: 2 in, 2 out]
              n67 = property on="TX_MIN_GAIN\nto\nTX_MAX_GAIN" class="DigNum (strict)"("Val(Sgnl)"=w134) -> ()  [unwired: 2 in, 2 out]
              n68 = invoke class="BBoxOneAPI" method="getAAKitList"(reference=w178, error in=w177, "sn"=w144) -> (reference out=w188:refnum<k24>, error out=w187:errorcluster, "getAAKitList"=w158:string[])  [unwired: 1 in, 1 out]
              "getAAKitList" <- w158
              n69 = Index String Array(1:"Target AAKit Index", 2:w158) -> (0:w155:string)  [unwired: 1 in]
              "Target AAKit Name" <- w155
              n70 = invoke class="BBoxOneAPI" method="selectAAKit"(reference=w188, error in=w187, "AAKitName"=w155, "sn"=w144) -> (reference out=w167:refnum<k24>, error out=w166:errorcluster, "selectAAKit"=→"selectAAKit":i32)  [unwired: 1 in, 2 out]
              n71 = invoke class="BBoxOneAPI" method="Get_All_BeamPattern_by_BeamType"(reference=w167, error in=w166, "mode"=1, "beam_type"=0, "sn"=w144) -> (reference out=w182:refnum<k24>, error out=w181:errorcluster, "Get_All_BeamPattern_by_BeamType"=→"TX Beam Table":string[][])  [unwired: 1 in, 3 out]
              n72 = invoke class="BBoxOneAPI" method="Get_All_BeamPattern_by_BeamType"(reference=w182, error in=w181, "mode"=2, "beam_type"=0, "sn"=w144) -> (reference out=w157:refnum<k24>, error out=w156:errorcluster, "Get_All_BeamPattern_by_BeamType"=→"RX Beam Table":string[][])  [unwired: 1 in, 3 out]
            }
            frame 3 {
            }
            frame 99 {
            }
          }
        }
      }
      event "TX Beam Pattern": Value Change {
        n73 = event-data() -> ()  [unwired: 1 in, 6 out]
        n74 = property on="Target SN" class="Str"(error in=w203) -> (error out=w202:errorcluster, "Value"=w204:string)  [unwired: 1 in, 1 out]
        n75 = invoke class="BBoxOneAPI" method="Set_BeamPattern_Config"(reference=w223, error in=w202, "beamId"="TX beamId :\nRange from\n1 to 64", "mode"=1, "db"="TX_MIN_GAIN\nto\nTX_MAX_GAIN", "theta"="TX Theta \nRange from\n0 to 45", "phi"="TX Phi :\nRange from\n0 to 359", "sn"=w204) -> (reference out=w221:refnum<k24>, error out=w222:errorcluster, "Set_BeamPattern_Config"=→"TX Store Beam Return":i32)  [unwired: 1 in, 6 out]
        n76 = invoke class="BBoxOneAPI" method="Get_All_BeamPattern_by_BeamType"(reference=w221, error in=w222, "mode"=1, "beam_type"=0, "sn"=w204) -> (reference out=w218:refnum<k24>, error out=w217:errorcluster, "Get_All_BeamPattern_by_BeamType"=w207:string[][])  [unwired: 1 in, 3 out]
        n77 = property on="TX Beam Table" class="Arr (strict)"("Value"=w207) -> ()  [unwired: 2 in, 2 out]
        n78 = invoke class="BBoxOneAPI" method="Get_All_BeamPattern_by_BeamType"(reference=w218, error in=w217, "mode"=2, "beam_type"=0, "sn"=w204) -> (reference out=w214:refnum<k24>, error out=w213:errorcluster, "Get_All_BeamPattern_by_BeamType"=w206:string[][])  [unwired: 1 in, 3 out]
        n79 = property on="RX Beam Table" class="Arr (strict)"("Value"=w206) -> ()  [unwired: 2 in, 2 out]
      }
      event "RX Beam Pattern": Value Change {
        n80 = event-data() -> ()  [unwired: 1 in, 6 out]
        n81 = property on="Target SN" class="Str"(error in=w227) -> (error out=w226:errorcluster, "Value"=w228:string)  [unwired: 1 in, 1 out]
        n82 = invoke class="BBoxOneAPI" method="Set_BeamPattern_Config"(reference=w247, error in=w226, "beamId"="RX beamId :\nRange from\n1 to 64", "mode"=2, "db"="RX_MIN_GAIN\nto\nRX_MAX_GAIN", "theta"="RX Theta \nRange from\n0 to 45", "phi"="RX Phi :\nRange from\n0 to 359", "sn"=w228) -> (reference out=w245:refnum<k24>, error out=w246:errorcluster, "Set_BeamPattern_Config"=→"RX Store Beam Return":i32)  [unwired: 1 in, 6 out]
        n83 = invoke class="BBoxOneAPI" method="Get_All_BeamPattern_by_BeamType"(reference=w245, error in=w246, "mode"=1, "beam_type"=0, "sn"=w228) -> (reference out=w242:refnum<k24>, error out=w241:errorcluster, "Get_All_BeamPattern_by_BeamType"=w231:string[][])  [unwired: 1 in, 3 out]
        n84 = property on="TX Beam Table" class="Arr (strict)"("Value"=w231) -> ()  [unwired: 2 in, 2 out]
        n85 = invoke class="BBoxOneAPI" method="Get_All_BeamPattern_by_BeamType"(reference=w242, error in=w241, "mode"=2, "beam_type"=0, "sn"=w228) -> (reference out=w238:refnum<k24>, error out=w237:errorcluster, "Get_All_BeamPattern_by_BeamType"=w230:string[][])  [unwired: 1 in, 3 out]
        n86 = property on="RX Beam Table" class="Arr (strict)"("Value"=w230) -> ()  [unwired: 2 in, 2 out]
      }
      event "Program Stop": Value Change {
        n87 = event-data() -> ()  [unwired: 1 in, 6 out]
        n88 = property on="checkCaliTableLocation" class="Bool (strict)"(error in=w251, "Val(Sgnl)"=FALSE ("Value (Signaling)")) -> (error out=w249:errorcluster)  [unwired: 1 in, 1 out]
      }
    }
  }
  n89 = Close Reference(reference=w8, error in (no error)=w7) -> ()  [unwired: 1 out]
